vi "Send Software Trigger.vi"(8 "error in (no error)":errorcluster {"code" format="%.0x"}, 11 "instrument handle":refnum<k15>) -> (0 "error out":errorcluster {"code" format="%.0x"}, 3 "instrument handle out":refnum<k15>)   [LabVIEW 2009, in "Keysight XSAn.lvlib"]
doc: "This function generates a software trigger.\n\nSupported Models: All supported"
uses:
  <instrlib>/Keysight XSAn/Keysight XSAn.lvlib
  AgXSAn.dll
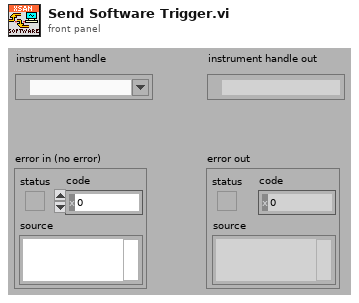
[diagram p1: front panel]
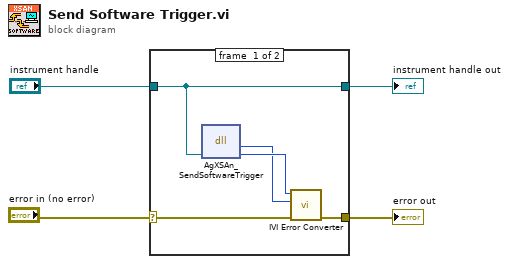
[diagram p0: block diagram]
diagram:
  n1 = case shown="No Error" "error in (no error)" {
    selector: "error in (no error)" -> [w7 w11]
    tunnel: [w8 w11] -> w3
    tunnel: "instrument handle" -> [w5 w10]
    tunnel: [w5 w10] -> w1
    frame #0 {
      n2 = dll-call lib="AgXSAn**.dll" fn="AgXSAn_SendSoftwareTrigger" ("LabVIEW:IviSpecAn_SendSoftwareTrigger")("instrument handle"=w5) -> ("Status"=w6:i32, "instrument handle"=w9:u32)  [unwired: 3 in, 2 out]
      n3 = call <instrlib>:"IVI Error Converter.vi"("error in (no error)"=w7, "IVI error code (0)"=w6, "instrument handle"=w9) -> ("error out"=w8:errorcluster)  [unwired: 7 in, 1 out]
    }
    frame #1 {
    }
  }
  "error out" <- w3
  "instrument handle out" <- w1
